vi "Launch Event Handle.vi"(8 "error in (no error)":errorcluster, 11 "QMenu Class in":refnum<class "QMenu Class.lvclass">) -> (0 "error out":errorcluster, 3 "QMenu Class out":refnum<class "QMenu Class.lvclass">)   [LabVIEW 2020, in "QTab.lvlib" / "QMenu Class.lvclass"]
uses:
  QMenu Class.lvclass
  QMenu Class.lvclass/QMenu Class.ctl
  Event Handle Dispatcher.vi
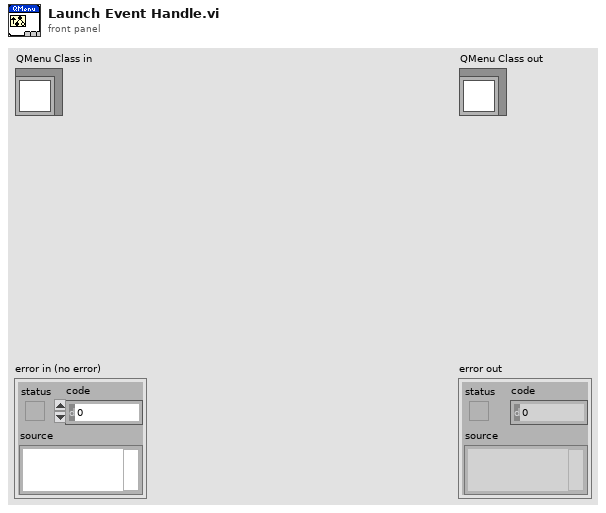
[diagram p1: front panel]
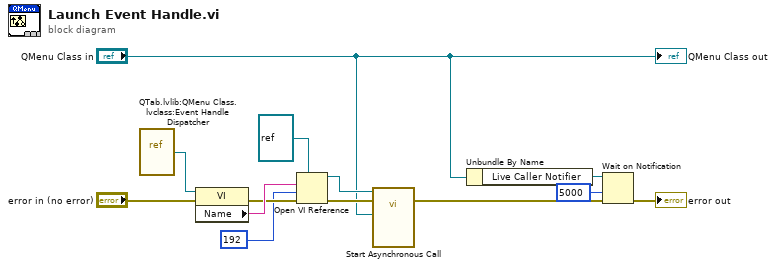
[diagram p0: block diagram]
diagram:
  n1 = vi-ref "QTab.lvlib:QMenu Class.lvclass:Event Handle Dispatcher.vi"() -> (w8:refnum<vi>)
  n2 = property class="VI"(reference=w8, error in="error in (no error)") -> (error out=w11:errorcluster, "Name"=w12:string)  [unwired: 1 out]
  n3 = Open VI Reference(type specifier VI Refnum (for type only)=refnum<vi> refnum, vi path=w12, options=192, error in (no error)=w11) -> (vi reference=w6:refnum<vi>, error out=w7:errorcluster)  [unwired: 2 in]
  n4 = call-by-ref "Start Asynchronous Call"(reference=w6, error in=w7, "MenuTab Class in"="QMenu Class in") -> (error out=w4:errorcluster)  [unwired: 10 in, 2 out]
  n5 = Unbundle By Name("QMenu Class in") -> ("Live Caller Notifier"=w3:refnum<notifier>)
  n6 = Wait on Notification(notifier=w3, timeout in ms (-1)=5000, error in (no error)=w4) -> (error out=→"error out":errorcluster)  [unwired: 1 in, 3 out]
  "QMenu Class out" <- "QMenu Class in"
